vi "Get Step Name.vi"(8 "error in (no error)":errorcluster, 11 "Step in":refnum<class "Step.lvclass">) -> (0 "error out":errorcluster, 2 "Step Name":string, 3 "Step out":refnum<class "Step.lvclass">)   [LabVIEW 2020, in "Tester.lvlib" / "Step.lvclass"]
uses:
  Step.lvclass
  <vilib>/regexp/Match Regular Expression.xnode
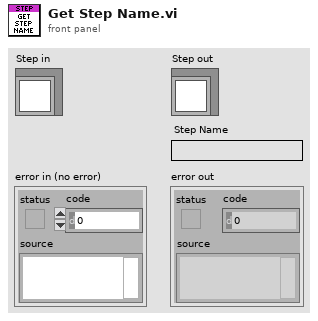
[diagram p1: front panel]
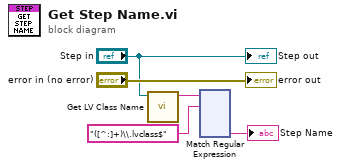
[diagram p0: block diagram]
diagram:
  n1 = call <vilib>:"Get LV Class Name.vi"("object"="Step in") -> ("class name"=w3:string)  [unwired: 9 in, 1 out]
  n2 = xnode "Match Regular Expression"("input string"=w3, "regular expression"="([^:]+)\\.lvclass$") -> ("submatch 1"=→"Step Name":string)  [unwired: 4 in, 5 out]
  "error out" <- "error in (no error)"
  "Step out" <- "Step in"
